vi "Clear All Memory Blocks.vi"   [LabVIEW 2010, in "Current Value Table.lvlib"]
doc: "This clears all memory blocks. New data types should be added to this VI."
uses:
  Current Value Table.lvlib
  Type Defs/Memory Commands.ctl
  DataTypes/Array of String_Memory Block.vi
  DataTypes/Array of Boolean_Memory Block.vi
  DataTypes/Array of Single_Memory Block.vi
  DataTypes/Array of Double_Memory Block.vi
  DataTypes/Array of I8_Memory Block.vi
  DataTypes/Array of I16_Memory Block.vi
  DataTypes/Array of I32_Memory Block.vi
  DataTypes/Array of I64_Memory Block.vi
  DataTypes/Array of U64_Memory Block.vi
  DataTypes/Array of U32_Memory Block.vi
  DataTypes/Array of U16_Memory Block.vi
  DataTypes/Array of U8_Memory Block.vi
  DataTypes/Boolean_Memory Block.vi
  DataTypes/String_Memory Block.vi
  DataTypes/U8_Memory Block.vi
  DataTypes/U16_Memory Block.vi
  DataTypes/U32_Memory Block.vi
  DataTypes/U64_Memory Block.vi
  DataTypes/I8_Memory Block.vi
  DataTypes/I16_Memory Block.vi
  DataTypes/I32_Memory Block.vi
  DataTypes/I64_Memory Block.vi
  DataTypes/Single_Memory Block.vi
  DataTypes/Double_Memory Block.vi
types:
  T1 = typedef "Current Value Table.lvlib/Memory Commands.ctl" = enum16{"Init", "Add Data", "Read", "Read Group", "Read All", "Write", "Write Group", "Get Size"}
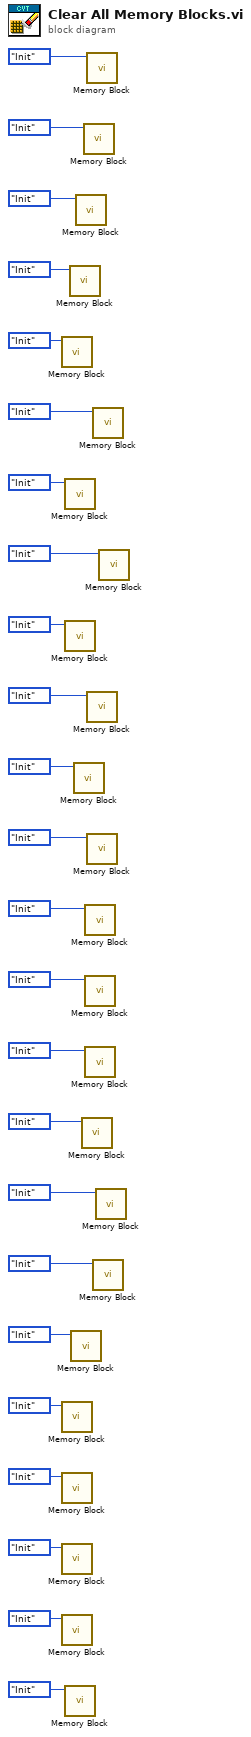
[diagram p0: block diagram]
diagram:
  n1 = call-poly "Memory Block.vi"("Method"=Memory_Commands."Init") -> ()  [unwired: 8 in, 3 out]
  n2 = call-poly "Memory Block.vi"("Method"=Memory_Commands."Init") -> ()  [unwired: 8 in, 3 out]
  n3 = call-poly "Memory Block.vi"("Method"=Memory_Commands."Init") -> ()  [unwired: 8 in, 3 out]
  n4 = call-poly "Memory Block.vi"("Method"=Memory_Commands."Init") -> ()  [unwired: 8 in, 3 out]
  n5 = call-poly "Memory Block.vi"("Method"=Memory_Commands."Init") -> ()  [unwired: 8 in, 3 out]
  n6 = call-poly "Memory Block.vi"("Method"=Memory_Commands."Init") -> ()  [unwired: 8 in, 3 out]
  n7 = call-poly "Memory Block.vi"("Method"=Memory_Commands."Init") -> ()  [unwired: 8 in, 3 out]
  n8 = call-poly "Memory Block.vi"("Method"=Memory_Commands."Init") -> ()  [unwired: 8 in, 3 out]
  n9 = call-poly "Memory Block.vi"("Method"=Memory_Commands."Init") -> ()  [unwired: 8 in, 3 out]
  n10 = call-poly "Memory Block.vi"("Method"=Memory_Commands."Init") -> ()  [unwired: 8 in, 3 out]
  n11 = call-poly "Memory Block.vi"("Method"=Memory_Commands."Init") -> ()  [unwired: 8 in, 3 out]
  n12 = call-poly "Memory Block.vi"("Method"=Memory_Commands."Init") -> ()  [unwired: 8 in, 3 out]
  n13 = call-poly "Memory Block.vi"("Method"=Memory_Commands."Init") -> ()  [unwired: 8 in, 3 out]
  n14 = call-poly "Memory Block.vi"("Method"=Memory_Commands."Init") -> ()  [unwired: 8 in, 3 out]
  n15 = call-poly "Memory Block.vi"("Method"=Memory_Commands."Init") -> ()  [unwired: 8 in, 3 out]
  n16 = call-poly "Memory Block.vi"("Method"=Memory_Commands."Init") -> ()  [unwired: 8 in, 3 out]
  n17 = call-poly "Memory Block.vi"("Method"=Memory_Commands."Init") -> ()  [unwired: 8 in, 3 out]
  n18 = call-poly "Memory Block.vi"("Method"=Memory_Commands."Init") -> ()  [unwired: 8 in, 3 out]
  n19 = call-poly "Memory Block.vi"("Method"=Memory_Commands."Init") -> ()  [unwired: 8 in, 3 out]
  n20 = call-poly "Memory Block.vi"("Method"=Memory_Commands."Init") -> ()  [unwired: 8 in, 3 out]
  n21 = call-poly "Memory Block.vi"("Method"=Memory_Commands."Init") -> ()  [unwired: 8 in, 3 out]
  n22 = call-poly "Memory Block.vi"("Method"=Memory_Commands."Init") -> ()  [unwired: 8 in, 3 out]
  n23 = call-poly "Memory Block.vi"("Method"=Memory_Commands."Init") -> ()  [unwired: 8 in, 3 out]
  n24 = call-poly "Memory Block.vi"("Method"=Memory_Commands."Init") -> ()  [unwired: 8 in, 3 out]
